vi "Digital Input Read Example.vi"() -> ()   [LabVIEW 2020]
uses:
  g_industrial_cam/Camera/Camera.lvclass/Camera.ctl
  g_industrial_cam/Camera/Set Value (String).vi
  g_industrial_cam/Camera/Get Value (Boolean).vi
  g_industrial_cam/Camera/GetSetTrigger.vi
  g_industrial_cam/Camera/GetSetStringValue.vi
  g_industrial_cam/Camera/GetSetBooleanValue.vi
  g_industrial_cam/Camera/Check Not Disconnected.vi
  <vilib>/Utility/error.llb/Error Cluster From Error Code.vi
  g_industrial_cam/Camera/Camera.lvclass
panel:
  in  "stop":bool
  out "Trigger Source Read Loop":i32
  out "Trigger Source Value":bool
  out "Current Trigger Source":string
  out "error out":errorcluster
  out "Trigger Sources":string[](array[string])
  # "This Example Lets You Read the Digital Level on a Physical Trigger Line"
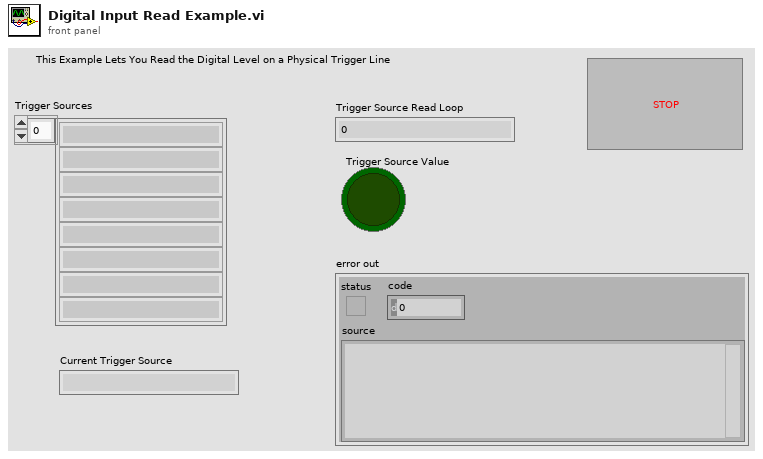
[diagram p1: front panel]
types:
  T1 = typedef "Device Enumeration.ctl" = cluster{"ID":string, "Protocol":string, "Vendor":string, "Model":string, "Serial":string, "Address":string}
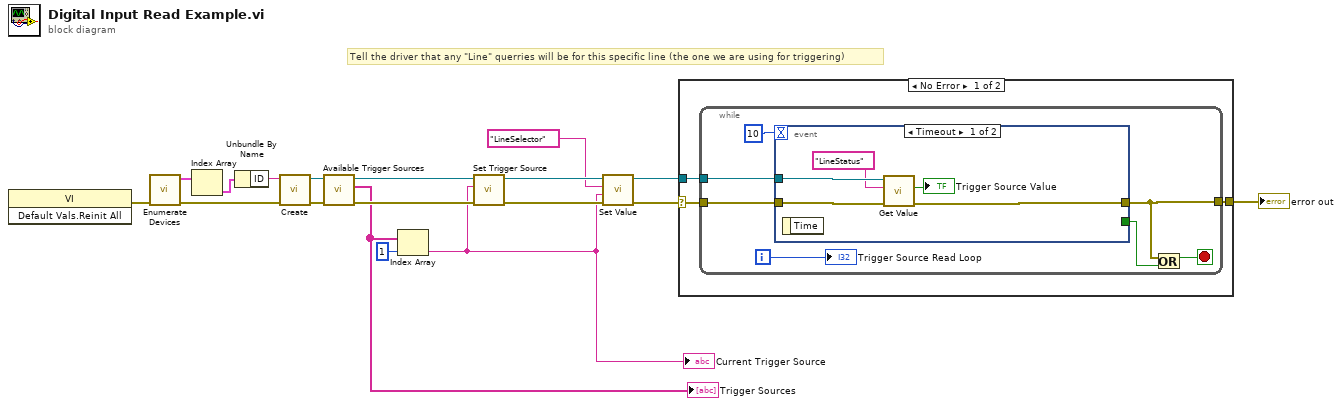
[diagram p0: block diagram]
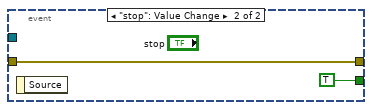
[diagram p2: hidden frame]
diagram:
  # "Tell the driver that any \"Line\" querries will be for this specific line (the one we are using for triggering)"
  n1 = invoke class="VI" method="Default Vals.Reinit All"() -> (error out=w8:errorcluster)  [unwired: 3 in, 2 out]
  n2 = call "Enumerate Devices.vi"("error in (no error)"=w8) -> ("error out"=w17:errorcluster, "Devices"=w18:T1[])  [unwired: 9 in]
  n3 = Index Array(array=w18) -> (element=w16:T1)  [unwired: 1 in]
  n4 = Unbundle By Name(w16) -> ("ID"=w15:string)
  n5 = call "Create.vi"("error in (no error)"=w17, "Identifier (ID, IP etc)"=w15) -> ("error out"=w6:errorcluster, "Camera"=w7:refnum<class "Camera.lvclass">)  [unwired: 8 in]
  n6 = call "Available Trigger Sources.vi"("error in (no error)"=w6, "Camera in"=w7) -> ("error out"=w5:errorcluster, "Available Trigger Sources"=w3:string[], "Camera"=w4:refnum<class "Camera.lvclass">)  [unwired: 7 in]
  "Trigger Sources" <- w3
  n7 = Index Array(array=w3, index=1) -> (element=w1:string)
  "Current Trigger Source" <- w1
  n8 = call "Set Trigger Source.vi"("error in (no error)"=w5, "Source"=w1, "Camera in"=w4) -> ("error out"=w14:errorcluster, "Camera"=w11:refnum<class "Camera.lvclass">)  [unwired: 7 in]
  n9 = call-poly "Set Value.vi"("error in (no error)"=w14, "Value"=w1, "Name"="LineSelector", "Camera in"=w11) -> ("error out"=w12:errorcluster, "Camera"=w10:refnum<class "Camera.lvclass">)  [unwired: 6 in]
  n10 = case shown="No Error" w12 {
    selector: w12 -> [w20 w36]
    tunnel: w10 -> [w21 _]
    tunnel: [w19 w36] -> w13
    frame No Error {
      n11 = while {
        tunnel: w21 -> [w28]
        tunnel: w20 -> [w26]
        tunnel: [w25] -> w19
        i -> [w24]
        stop <- w23 stop-if-true
        n12 = event shown="[0] Timeout" {
          selector: _ -> [_ _]
          dyn-events: _ -> [_ _]
          timeout: 10 -> [_ _]
          tunnel: w28 -> [w33 _]
          tunnel: [w32 w35] -> w25
          tunnel: w26 -> [w31 w35]
          tunnel: [_ TRUE] -> w22
          event Timeout {
            n13 = event-data() -> ()  [unwired: 1 in, 1 out]
            n14 = call-poly "Get Value.vi"("error in (no error)"=w31, "Name"="LineStatus", "Camera in"=w33) -> ("error out"=w32:errorcluster, "Value"=→"Trigger Source Value":bool)  [unwired: 6 in, 1 out]
          }
          event "stop": Value Change {
            n15 = event-data() -> ()  [unwired: 1 in, 1 out]
          }
        }
        n16 = Or(x=w25, y=w22) -> (x .or. y?=w23:bool)
        "Trigger Source Read Loop" <- w24
      }
    }
    frame Error {
    }
  }
  "error out" <- w13
